vi "AImotive UDP Receivier.vi"(8 "error in (no error)":errorcluster, 10 "stop":bool, 11 "receiver port":u16=61557) -> (0 "error out":errorcluster, 2 "Number Squared Array":dbl[](array[numeric]))   [LabVIEW 2019]
doc: "The UDP protocol differs from TCP in that there is no error-checking with the packets of information that are sent, and thus no guarantee whatsoever that an intended recipient will actually receive a given piece of data.\n\nUDP does offer the ability to \"broadcast\" data across a network--simply specify an IP Address of all ones (255.255.255.255) to attempt to broadcast information network-wide. Keep in mind that routers and other network hardware will generally refuse to forward the broadcast beyond certain points, so the extent of the broadcast will in practice be limited."
panel:
  out "Current Value":dbl
  # "Overview: Listens for data from UDP - Sender.vi on ports in UDP Ports to Check array. Returns received data in graphical and array form and logs the results to disc.\n\nInstructions:\n1. Ensure UDP - Sender.vi is already running.\n2. Run the VI.\n3. Click Start to start the test."
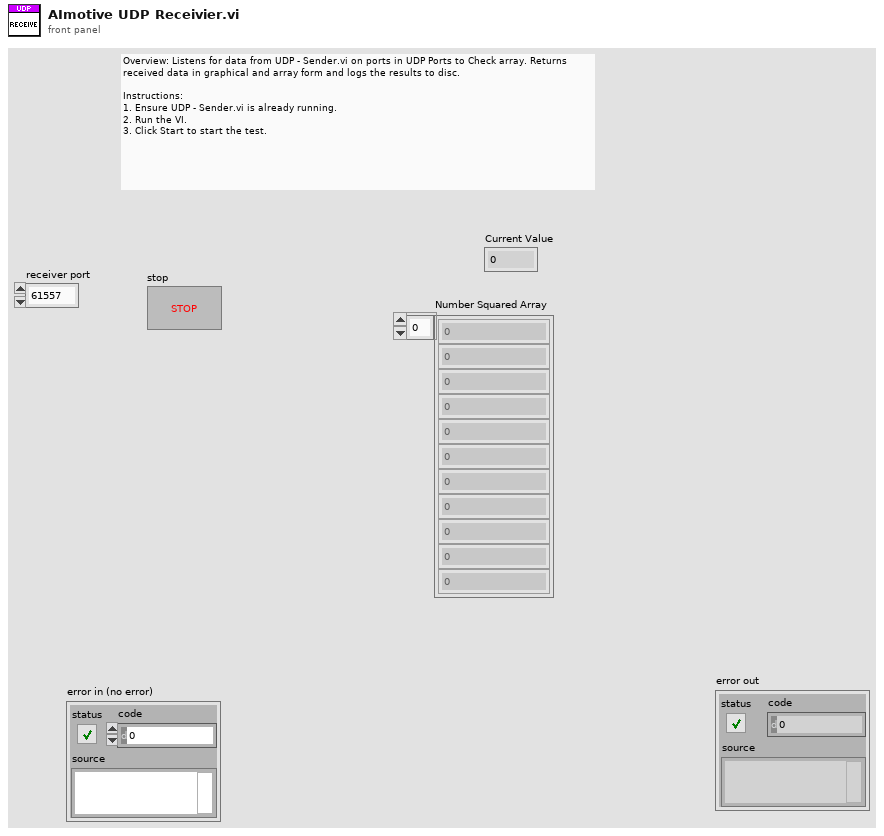
[diagram p1: front panel]
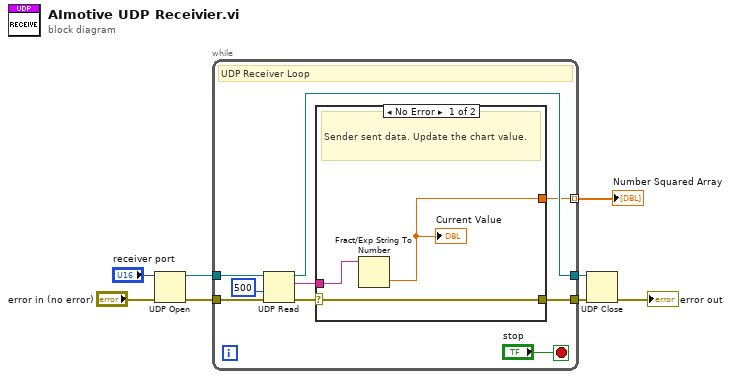
[diagram p0: block diagram]
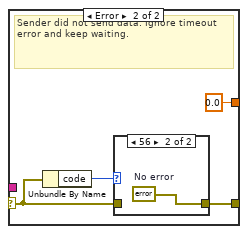
[diagram p2: hidden frame]
diagram:
  n1 = UDP Open(8:"error in (no error)", 11:"receiver port") -> (port=w4:refnum<k16>, 0:w5:errorcluster)  [unwired: 3 in, 1 out]
  n2 = while {
    tunnel: w4 -> [w17]
    tunnel: [w11] -> w7
    tunnel: w5 -> [w16]
    tunnel: [w12] -> w6
    tunnel: [w9] -> w1 mode=indexing
    stop <- "stop" stop-if-true
    # "UDP Receiver Loop"
    n3 = UDP Read(connection ID=w17, timeout ms (25000)=500, 8:w16) -> (data out=w14:string, error out=w13:errorcluster, 3:w11:refnum<k16>)  [unwired: 3 out]
    n4 = case shown="No Error" w13 {
      selector: w13 -> [w19 w23]
      tunnel: w14 -> [w20 _]
      tunnel: [w19 w22] -> w12
      tunnel: [w18 0.0] -> w9
      frame No Error {
        # "Sender sent data. Update the chart value."
        n5 = Fract/Exp String To Number(string=w20) -> (number=w18:dbl)  [unwired: 3 in, 1 out]
        "Current Value" <- w18
      }
      frame Error {
        # "Sender did not send data. Ignore timeout error and keep waiting."
        n6 = Unbundle By Name(w23) -> ("code"=w24:i32)
        n7 = case shown="56" w24 {
          tunnel: w23 -> [w25 _]
          tunnel: [w25 w26] -> w22
          frame Default {
          }
          frame 56 {
            w26 = errorcluster {"status"=FALSE, "code"=0, "source"=""}  # No error
          }
        }
      }
    }
  }
  "Number Squared Array" <- w1
  n8 = UDP Close(connection ID=w7, 8:w6) -> (error out=→"error out":errorcluster)  [unwired: 1 out]
